vi "set_ylim.vi"(6 "ylim":dbl[](array[numeric]), 8 "error in":errorcluster, 11 "figure (in)":refnum<vi>) -> (0 "error out":errorcluster, 3 "figure (out)":refnum<vi>)   [LabVIEW 2017]
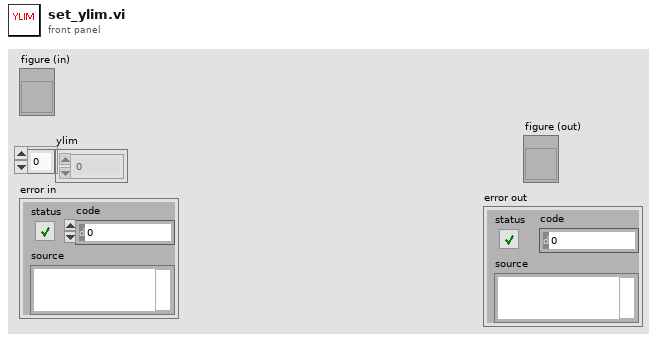
[diagram p1: front panel]
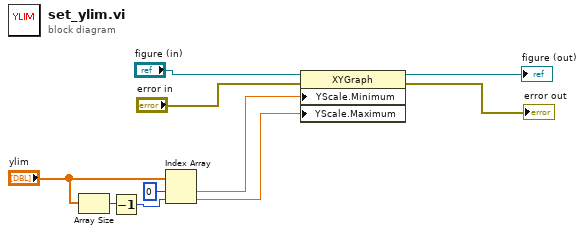
[diagram p0: block diagram]
diagram:
  n1 = Array Size(array="ylim") -> (size(s)=w2:i32)
  n2 = Decrement(x=w2) -> (x-1=w1:i32)
  n3 = Index Array(array="ylim", index #1=0 ("index"), index #2=w1) -> (element #1=w6:dbl, element #2=w5:dbl)
  n4 = property on="Property Node" class="XYGraph"(reference="figure (in)", error in="error in", "YScale.Minimum"=w6, "YScale.Maximum"=w5) -> (reference out=→"figure (out)":refnum<vi>, error out=→"error out":errorcluster)
